vi "Opdracht_1_Pakgetallenmetlengte8eruit.vi"(10 "array w/ subset deleted":string[](array[string])) -> (1 "Array":string[](array[string]), 3 "N":dbl[](array[numeric]))   [LabVIEW 2018]
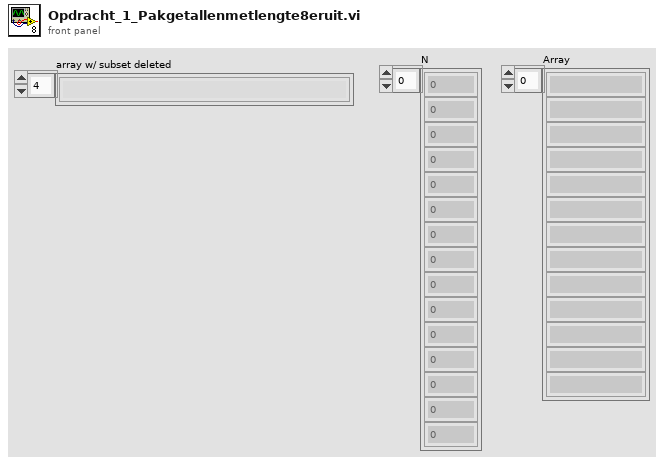
[diagram p1: front panel]
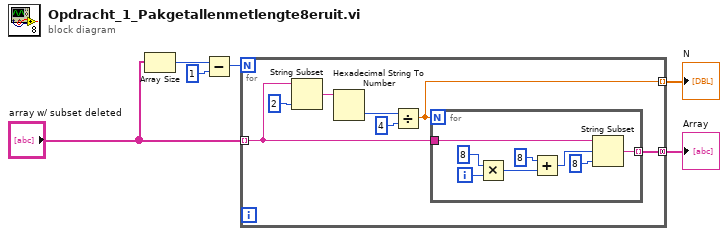
[diagram p0: block diagram]
diagram:
  n1 = Array Size(array="array w/ subset deleted") -> (size(s)=w4:i32)
  n2 = Subtract(x=w4, y=1) -> (x-y=w2:i32)
  n3 = for {
    N: w2 -> [_]
    tunnel: "array w/ subset deleted" -> [w7] mode=indexing
    tunnel: [w9] -> w1 mode=concatenating
    tunnel: [w8] -> w5 mode=indexing
    n4 = String Subset(string=w7, length (rest)=2 ("length (rest)")) -> (substring=w10:string)  [unwired: 1 in]
    n5 = Hexadecimal String To Number(string=w10) -> (number=w11:u32)  [unwired: 2 in, 1 out]
    n6 = Divide(x=w11, y=u32 4) -> (x/y=w8:dbl)
    n7 = for {
      N: w8 -> [_]
      tunnel: w7 -> [w14]
      tunnel: [w20] -> w9 mode=indexing
      i -> [w19]
      n8 = Multiply(x=8 ("offset (0)"), y=w19) -> (x*y=w17:i32)
      n9 = Add(x=8, y=w17) -> (x+y=w15:i32)
      n10 = String Subset(string=w14, offset (0)=w15, length (rest)=8 ("length (rest)")) -> (substring=w20:string)
    }
  }
  "N" <- w5
  "Array" <- w1
